vi "Packet Transmitter Global.vi"(8 "Action":T2=enum."Enqueue for Send", 10 "Data In":u8[](array[numeric]), 11 "Packet Type":T1) -> (1 "notifier out":refnum<notifier>)   [LabVIEW 2015]
uses:
  Packet Transmitter Action.ctl
  Control Packet Type.ctl
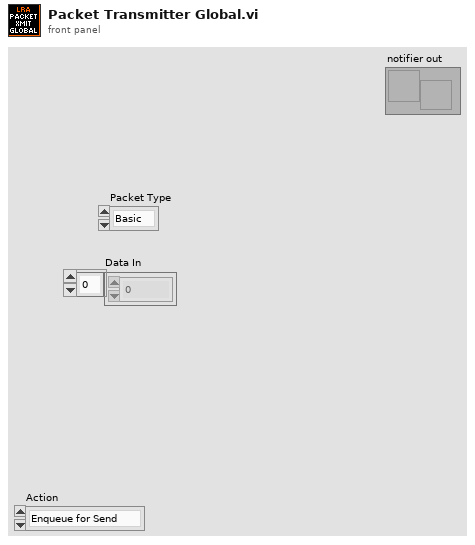
[diagram p1: front panel]
types:
  T1 = typedef "Control Packet Type.ctl" = enum8{"Basic"}
  T2 = typedef "Packet Transmitter Action.ctl" = enum16{"Initialize", "Enqueue for Send", "Retrieve for Send"}
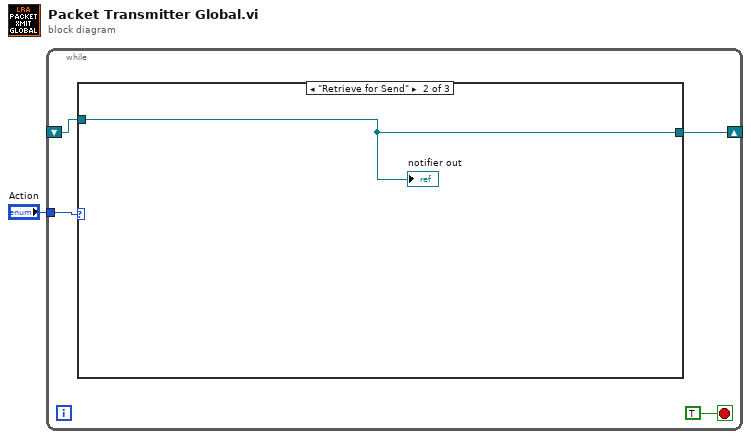
[diagram p0: block diagram]
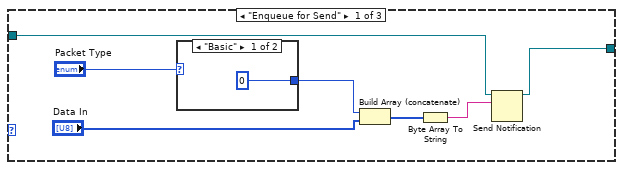
[diagram p2: hidden frame]
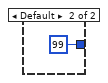
[diagram p3: hidden frame]
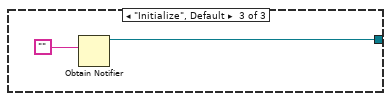
[diagram p4: hidden frame]
diagram:
  n1 = while {
    tunnel: "Action" -> [w5]
    shift-right: [w3] -> _
    shift-left: _ -> [w2]
    stop <- TRUE stop-if-true
    n2 = case shown="\"Retrieve for Send\"" w5 {
      tunnel: [w7 w15 w17] -> w3
      tunnel: w2 -> [w6 w15 _]
      frame "Enqueue for Send" {
        n3 = case shown="\"Basic\"" "Packet Type" {
          tunnel: [u8 0 u8 99] -> w11
          frame "Basic" {
          }
          frame Default {
          }
        }
        n4 = Build Array (concatenate)(w11, "Data In") -> (w9:u8[])
        n5 = Byte Array To String(unsigned byte array=w9) -> (string=w8:string)
        n6 = Send Notification(notification=w8, notifier=w6) -> (notifier out=w7:refnum<notifier>)  [unwired: 1 in, 1 out]
      }
      frame "Retrieve for Send" {
        "notifier out" <- w15
      }
      frame "Initialize", Default {
        n7 = Obtain Notifier(notification data type="") -> (notifier out=w17:refnum<notifier>)  [unwired: 3 in, 2 out]
      }
    }
  }
